vi "ManualUpload.vi"() -> ()   [LabVIEW 2020]
uses:
  Keithley_Subs/CapacitanceInfos.ctl
  Keithley_Subs/CapacitanceRecord.ctl
  <vilib>/Utility/file.llb/Read Delimited Spreadsheet (DBL).vi
  <vilib>/httpClient/POSTBuffer.vi
  <vilib>/httpClient/LabVIEWHTTPClient.lvlib
panel:
  out "error out 2":errorcluster
  out "array":string[][](array[string])
  out "All Files in Dir":path[](array[path])
  in  "SideLength":dbl=1.0
  in  "Area":dbl=1.0
  in  "Cluster 3":T3={"Intercept Error"=0.0, "Slope Error"=0.0, "Intercept"=0.0, "Slope"=0.0, "DataType"="", "Current"=[], "Voltage"=[], "Capacitance"=0.0, "Area"=0.0, "SideLength"=0.0, "InfoCluster"={"Conductance"=0.0, "CapacitanceIV"=0.0, "Intercept"=0.0, "CapacitanceSW"=0.0, "Sum"=0.0, "CapacitanceInfos"=[], "CapacitancePhase"=0.0, "dC/dV"=0.0}, "TimeStep"=0.0, "Source"="ProbeStation"}
  out "error out":errorcluster
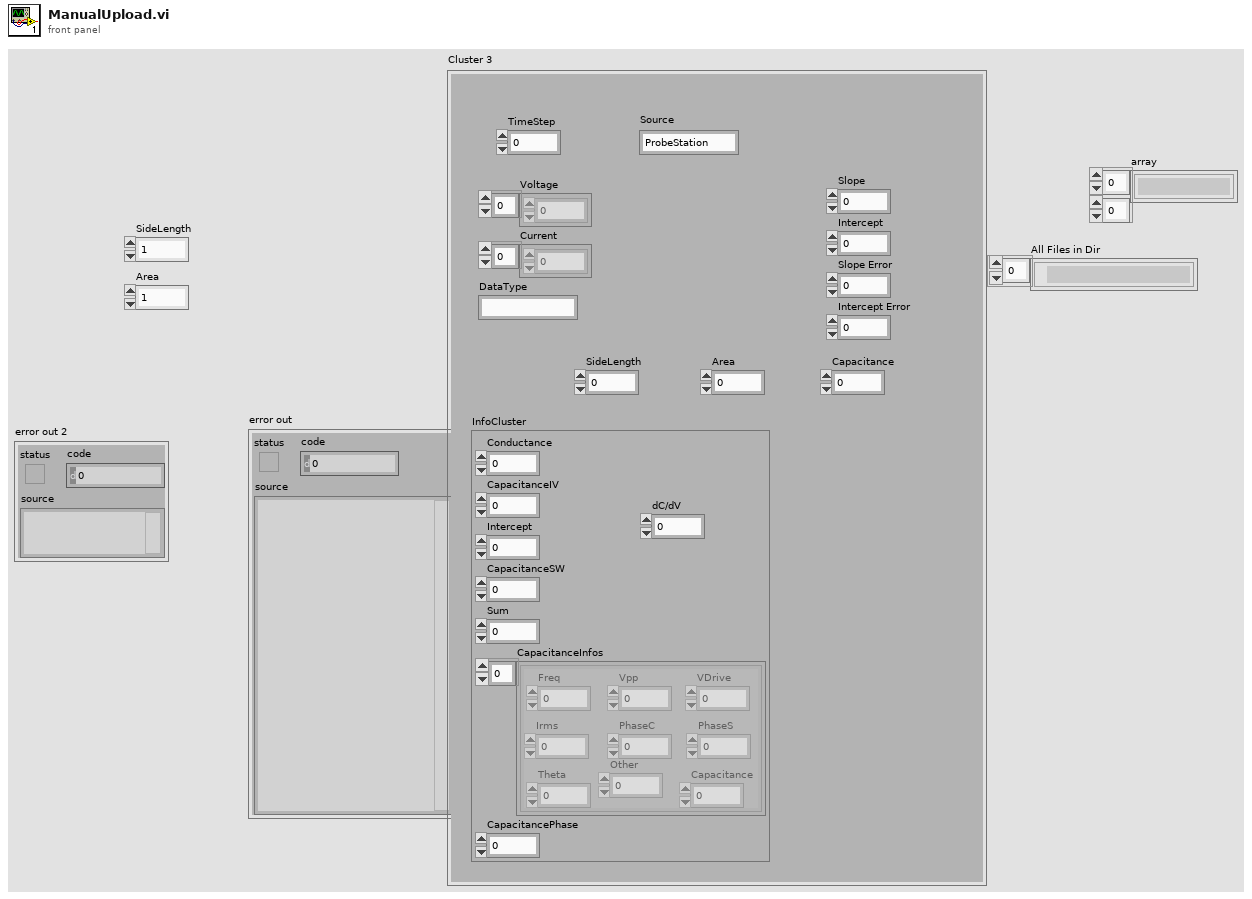
[diagram p1: front panel]
types:
  T1 = typedef "CapacitanceInfos.ctl" = cluster{"Conductance":dbl, "CapacitanceIV":dbl, "Intercept":dbl, "CapacitanceSW":dbl, "Sum":dbl, "CapacitanceInfos":T2[], "CapacitancePhase":dbl, "dC/dV":dbl}
  T2 = typedef "CapacitanceRecord.ctl" = cluster{"Freq":dbl, "Vpp":dbl, "PhaseS":dbl, "Irms":dbl, "PhaseC":dbl, "Theta":dbl, "VDrive":dbl, "Capacitance":dbl, "Other":dbl}
  T3 = cluster{"Intercept Error":dbl, "Slope Error":dbl, "Intercept":dbl, "Slope":dbl, "DataType":string, "Current":dbl[], "Voltage":dbl[], "Capacitance":dbl, "Area":dbl, "SideLength":dbl, "InfoCluster":T1, "TimeStep":dbl, "Source":string}
  T4 = typedef "LabVIEWHTTPClient.lvlib/ClientHandle.ctl" = refnum<k1>
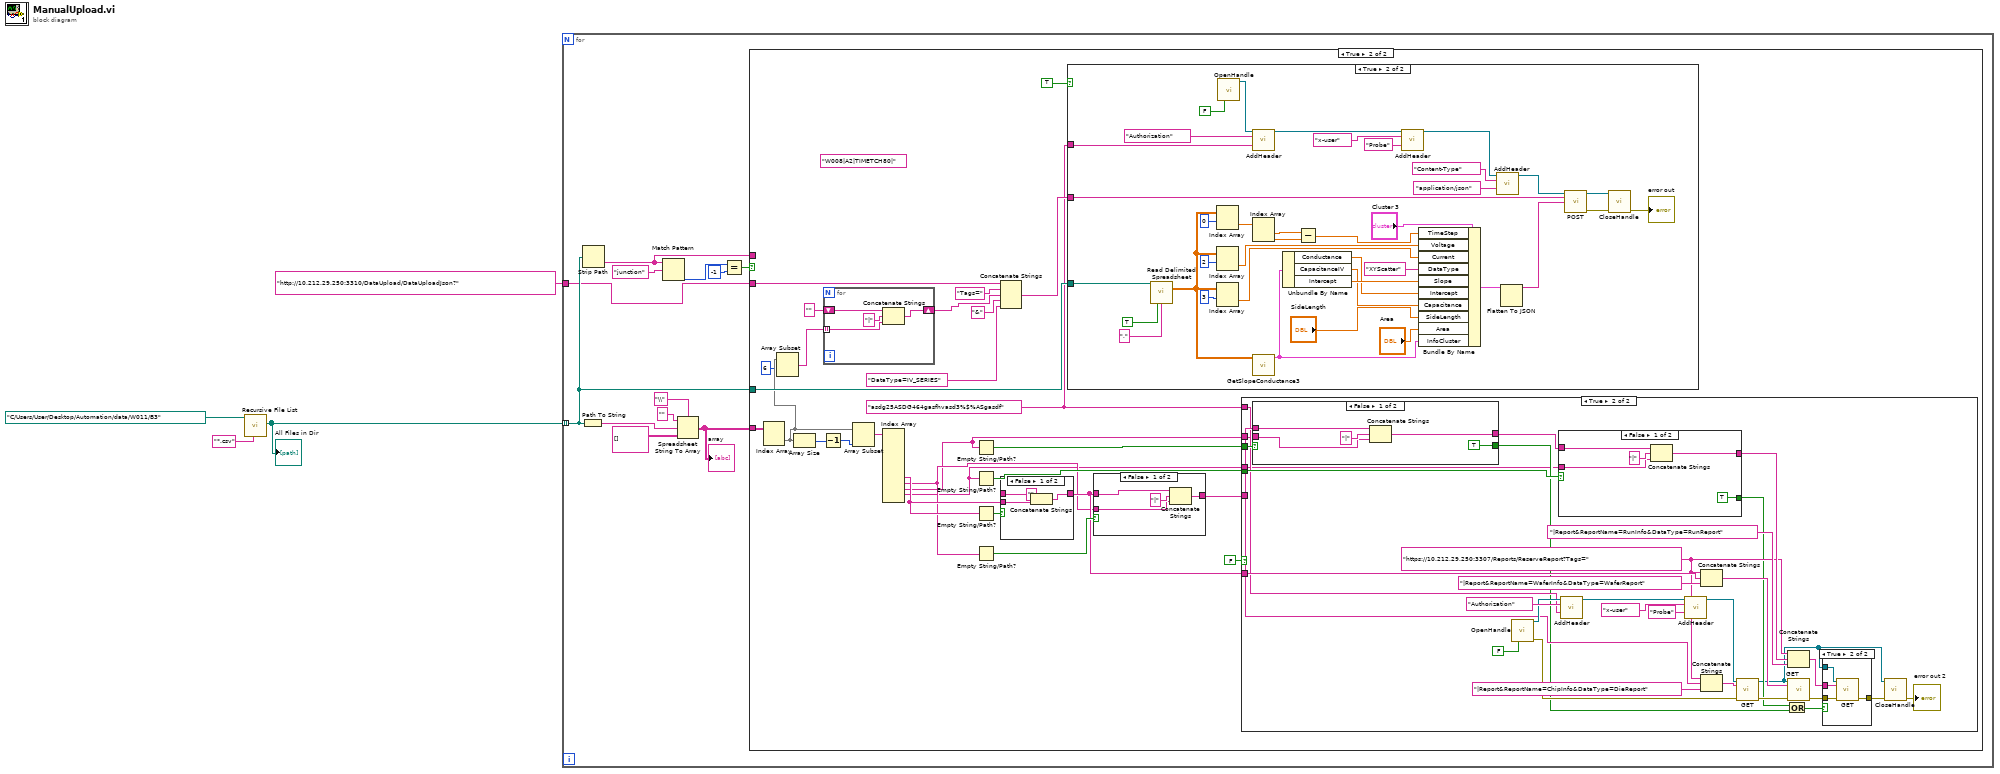
[diagram p0: block diagram]
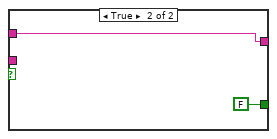
[diagram p5: hidden frame]
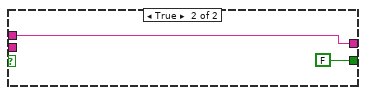
[diagram p6: hidden frame]
diagram:
  n1 = call <vilib>:"Recursive File List.vi"("pattern"="*.csv", "Folder Path"=path "C:/Users/User/Desktop/Automation/data/W011/B3" ("path")) -> ("All Files in Dir"=w2:path[])  [unwired: 5 in, 4 out]
  "All Files in Dir" <- w2
  n2 = for {
    tunnel: w2 -> [w14] mode=indexing
    tunnel: "http://10.212.29.250:3310/DataUpload/DataUploadJson?" ("input string") -> [w5]
    n3 = Path To String(path=w14) -> (string=w13:string)
    n4 = Strip Path(path=w14) -> (name=w16:string)  [unwired: 1 out]
    n5 = Match Pattern(string=w16, regular expression="junction") -> (offset past match=w9:i32)  [unwired: 1 in, 3 out]
    n6 = Spreadsheet String To Array(delimiter (Tab)="\\" ("search string/char (-)"), format string="", spreadsheet string=w13, array type (2D Dbl)=string[][] []) -> (array=w6:string[][])
    "array" <- w6
    n7 = Equal?(x=w9, y=-1) -> (x = y?=w7:bool)
    n8 = case shown="True" w7 {
      tunnel: w16 -> [_ _]
      tunnel: w14 -> [_ w45]
      tunnel: w5 -> [_ w44]
      tunnel: w6 -> [_ w38]
      frame False {
      }
      frame True {
        (unwired) "W008|A2|TIMETCH80|"
        w29 = "asdg25ASDG464gasfhvasd3%$%ASgasdf" ("value")
        n9 = Index Array(array=w38) -> (element=w20:string[])  [unwired: 2 in]
        n10 = Array Subset(array=w20, index=6) -> (w21:string[])  [unwired: 1 in]
        n11 = Array Size(array=w20) -> (size(s)=w27:i32)
        n12 = Decrement(x=w27) -> (x-1=w26:i32)
        n13 = for {
          shift-right: [w146] -> w17
          shift-left: "" -> [w145]
          tunnel: w21 -> [w144] mode=indexing
          n14 = Concatenate Strings(w145, "|" ("string"), w144) -> (w146:string)
        }
        n15 = Array Subset(array=w20, length=w26) -> (w28:string[])  [unwired: 1 in]
        n16 = Index Array(array=w28) -> (element #7=w25:string, element #8=w24:string, element #9=w23:string, element #10=w22:string)  [unwired: 11 in, 7 out]
        n17 = Empty String/Path?(string/path=w23) -> (empty?=w34:bool)
        n18 = Empty String/Path?(string/path=w22) -> (empty?=w33:bool)
        n19 = Empty String/Path?(string/path=w25) -> (empty?=w36:bool)
        n20 = Empty String/Path?(string/path=w24) -> (empty?=w35:bool)
        n21 = Concatenate Strings(w44, "Tags=" ("string"), w17, "&" ("string"), "DataType=IV_SERIES" ("string")) -> (w42:string)
        n22 = case shown="False" w36 {
          tunnel: "" -> [w142 w143]
          tunnel: [w141 w143] -> w32
          tunnel: w25 -> [w140 _]
          frame False {
            n23 = Concatenate Strings(w142, w140) -> (w141:string)
          }
          frame True {
          }
        }
        n24 = case shown="True" TRUE {
          tunnel: w45 -> [_ w110]
          tunnel: w42 -> [_ w103]
          tunnel: w29 -> [_ w97]
          frame False {
          }
          frame True {
            n25 = call-poly <vilib>:"Read Delimited Spreadsheet.vi"("file path (dialog if empty)"=w110, "transpose? (F)"=TRUE, "delimiter (\\t)"="," ("delimiter (\\t)")) -> ("all rows"=w112:dbl[][])  [unwired: 7 in, 5 out]
            n26 = Index Array(array=w112, index (row)=0) -> (element=w108:dbl[])  [unwired: 1 in]
            n27 = Index Array(array=w112, index (row)=2) -> (element=w131:dbl[])  [unwired: 1 in]
            n28 = Index Array(array=w112, index (row)=3) -> (element=w132:dbl[])  [unwired: 1 in]
            n29 = call <vilib>:"OpenHandle.vi"("verify server(true)"=FALSE) -> ("client handle out"=w98:T4)  [unwired: 13 in, 1 out]
            n30 = call <vilib>:"AddHeader.vi"("client handle"=w98, "header"="Authorization", "value"=w97) -> ("client handle out"=w123:T4)  [unwired: 11 in, 1 out]
            n31 = Index Array(array=w108) -> (element #1=w106:dbl, element #2=w107:dbl)  [unwired: 2 in]
            n32 = call "GetSlopeConductance3.vi"("Array in"=w112) -> ("InfoCluster"=w111:T1)  [unwired: 9 in, 1 out]
            n33 = Unbundle By Name(w111) -> ("Conductance"=w119:dbl, "CapacitanceIV"=w117:dbl, "Intercept"=w118:dbl)
            n34 = Subtract(x=w106, y=w107) -> (x-y=w105:dbl)
            n35 = call <vilib>:"AddHeader.vi"("client handle"=w123, "header"="x-user", "value"="Probe") -> ("client handle out"=w114:T4)  [unwired: 11 in, 1 out]
            n36 = Bundle By Name(cluster="Cluster 3", "TimeStep"=w105, "Voltage"=w131, "Current"=w132, "DataType"="XYScatter", "Slope"=w119, "Intercept"=w118, "Capacitance"=w117, "SideLength"="SideLength", "Area"="Area", "InfoCluster"=w111) -> (w134:T3)
            n37 = call <vilib>:"AddHeader.vi"("client handle"=w114, "header"="Content-Type", "value"="application/json") -> ("client handle out"=w113:T4)  [unwired: 11 in, 1 out]
            n38 = Flatten To JSON(anything=w134) -> (JSON string=w127:string)  [unwired: 2 in, 1 out]
            n39 = call-poly <vilib>:"POST.vi"("client handle"=w113, "url"=w103, "buffer"=w127) -> ("client handle out"=w100:T4, "error out"=w99:errorcluster)  [unwired: 9 in, 2 out]
            n40 = call <vilib>:"CloseHandle.vi"("client handle"=w100, "error in (no error)"=w99) -> ("error out"=→"error out":errorcluster)  [unwired: 13 in]
          }
        }
        n41 = case shown="False" w35 {
          tunnel: w32 -> [w138 w139]
          tunnel: [w137 w139] -> w31
          tunnel: w24 -> [w135 _]
          frame False {
            n42 = Concatenate Strings(w138, "|" ("string"), w135) -> (w137:string)
          }
          frame True {
          }
        }
        n43 = case shown="True" FALSE {
          tunnel: w34 -> [_ w68]
          tunnel: w33 -> [_ w67]
          tunnel: w32 -> [_ w55]
          tunnel: w31 -> [_ w54]
          tunnel: w29 -> [_ w53]
          tunnel: w23 -> [_ w47]
          tunnel: w22 -> [_ w46]
          frame False {
          }
          frame True {
            w52 = "https://10.212.29.250:3307/Reports/ReserveReport?Tags=" ("input string")
            n44 = case shown="False" w68 {
              tunnel: w54 -> [w94 w96]
              tunnel: [w93 w96] -> w66
              tunnel: w47 -> [w91 _]
              tunnel: [TRUE FALSE] -> w49
              frame False {
                n45 = Concatenate Strings(w94, "|" ("string"), w91) -> (w93:string)
              }
              frame True {
              }
            }
            n46 = call <vilib>:"OpenHandle.vi"("verify server(true)"=FALSE) -> ("client handle out"=w71:T4, "error out"=w76:errorcluster)  [unwired: 13 in]
            n47 = case shown="False" w67 {
              tunnel: w66 -> [w87 w89]
              tunnel: [w86 w89] -> w58
              tunnel: w46 -> [w84 _]
              tunnel: [TRUE FALSE] -> w50
              frame False {
                n48 = Concatenate Strings(w87, "|" ("string"), w84) -> (w86:string)
              }
              frame True {
              }
            }
            n49 = call <vilib>:"AddHeader.vi"("client handle"=w71, "header"="Authorization", "value"=w53) -> ("client handle out"=w75:T4)  [unwired: 11 in, 1 out]
            n50 = call <vilib>:"AddHeader.vi"("client handle"=w75, "header"="x-user", "value"="Probe") -> ("client handle out"=w64:T4)  [unwired: 11 in, 1 out]
            n51 = Concatenate Strings(w52, w55, "|Report&ReportName=WaferInfo&DataType=WaferReport" ("string")) -> (w61:string)
            n52 = Concatenate Strings(w52, w54, "|Report&ReportName=ChipInfo&DataType=DieReport" ("string")) -> (w69:string)
            n53 = call <vilib>:"GET.vi"("client handle"=w64, "url"=w69, "error in (no error)"=w76) -> ("client handle out"=w48:T4, "error out"=w62:errorcluster)  [unwired: 9 in, 2 out]
            n54 = Or(x=w50, y=w49) -> (x .or. y?=w51:bool)
            n55 = Concatenate Strings(w52, w58, "|Report&ReportName=RunInfo&DataType=RunReport" ("string")) -> (w59:string)
            n56 = call <vilib>:"GET.vi"("client handle"=w48, "url"=w61, "error in (no error)"=w62) -> ("error out"=w57:errorcluster)  [unwired: 9 in, 3 out]
            n57 = case shown="True" w51 {
              tunnel: w59 -> [_ w82]
              tunnel: w57 -> [w78 w81]
              tunnel: [w78 w80] -> w56
              tunnel: w48 -> [_ w79]
              frame False {
              }
              frame True {
                n58 = call <vilib>:"GET.vi"("client handle"=w79, "url"=w82, "error in (no error)"=w81) -> ("error out"=w80:errorcluster)  [unwired: 9 in, 3 out]
              }
            }
            n59 = call <vilib>:"CloseHandle.vi"("client handle"=w48, "error in (no error)"=w56) -> ("error out"=→"error out 2":errorcluster)  [unwired: 13 in]
          }
        }
      }
    }
  }
